vi "Q5_transfer_2_Z.vi"(3 "Qn":dbl[](array[numeric]), 4 "x":dbl format="%#_13g") -> (1 "y":dbl)   [LabVIEW 2015]
panel:
  out "x*y 2":dbl[](array[numeric])
  out "xk chain":dbl[](array[numeric])
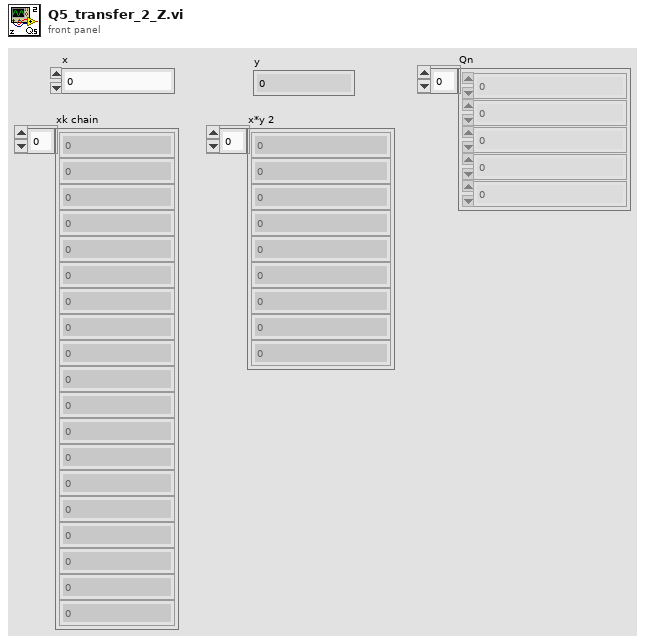
[diagram p1: front panel]
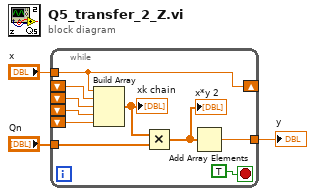
[diagram p0: block diagram]
diagram:
  n1 = while {
    tunnel: [w4] -> w3
    tunnel: "x" -> [w12]
    tunnel: "Qn" -> [w8]
    shift-right: [w12] -> _
    shift-left: _ -> [w11]
    shift-left: _ -> [w7]
    shift-left: _ -> [w6]
    shift-left: _ -> [w5]
    stop <- TRUE stop-if-true
    n2 = Build Array(w12, w11, w7, w6, w5) -> (w9:dbl[])
    "xk chain" <- w9
    n3 = Multiply(x=w9, y=w8) -> (x*y=w13:dbl[])
    "x*y 2" <- w13
    n4 = Add Array Elements(numeric array=w13) -> (sum=w4:dbl)
  }
  "y" <- w3
